vi "Update Status.vi"(8 "error in (no error)":errorcluster, 9 "Status":T1, 10 "Case":string, 11 "Icon Decorator V2 In":refnum<class "Icon Decorator V2.lvclass">) -> (0 "error out":errorcluster, 3 "Icon Decorator V2 Out":refnum<class "Icon Decorator V2.lvclass">)   [LabVIEW 2020, in "Icon Decorator V2.lvclass"]
uses:
  Icon Decorator V2.lvclass
  Result/Status.ctl
  Icon Decorator V2.lvclass/Icon Decorator V2.ctl
  Result/Result.lvlib
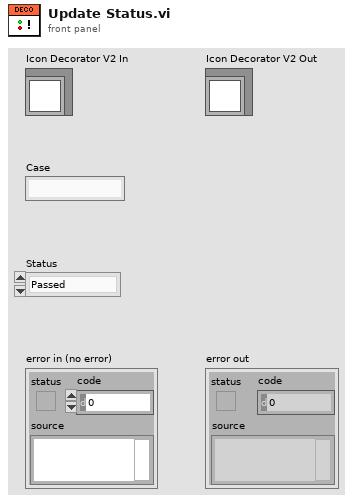
[diagram p1: front panel]
types:
  T1 = typedef "Result.lvlib/Status.ctl" = enum16{"Passed", "Failed", "Error", "Skipped", "Setup Error", "Broken", "Teardown Error"}
  T2 = typedef "ItemRef.ctl" = u64
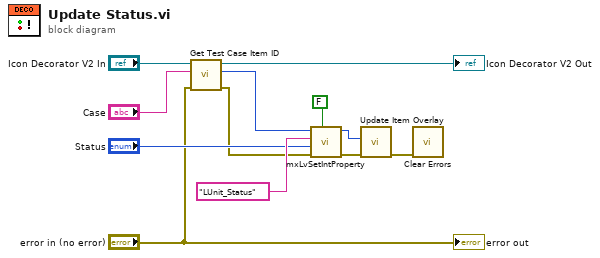
[diagram p0: block diagram]
diagram:
  n1 = call "Get Test Case Item ID.vi"("error in (no error)"="error in (no error)", "Test Case"="Case", "Icon Decorator V2 In"="Icon Decorator V2 In") -> ("error out"=w3:errorcluster, "ObjectItem"=w4:T2, "Icon Decorator V2 Out"=→"Icon Decorator V2 Out":refnum<class "Icon Decorator V2.lvclass">)  [unwired: 6 in]
  n2 = call <resource>:"mxLvSetIntProperty.vi"("Persist Property? (T)"=FALSE, "error in"=w3, "Value (0)"="Status", "Tag"="LUnit_Status", "Item"=w4) -> ("error out"=w8:errorcluster, "Item"=w9:T2)  [unwired: 5 in]
  n3 = call "Update Item Overlay.vi"("error in (no error)"=w8, "Item"=w9) -> ("error out"=w1:errorcluster)  [unwired: 9 in]
  n4 = call <vilib>:"Clear Errors.vi"("error in (no error)"=w1) -> ()  [unwired: 5 in, 2 out]
  "error out" <- "error in (no error)"
